vi "saveData.vi"(8 "error in (no error)":errorcluster, 11 "reference in":refnum<class "Devices Controller.lvclass">) -> (0 "error out":errorcluster, 3 "reference out":refnum<class "Devices Controller.lvclass">)   [LabVIEW 2016, in "Devices Controller.lvclass"]
uses:
  Devices Controller.lvclass
  APP/excelFile_class/fileType.ctl
  File Controller_llb/File Controller.lvclass
  APP/excelFile_class/excelFile.lvclass
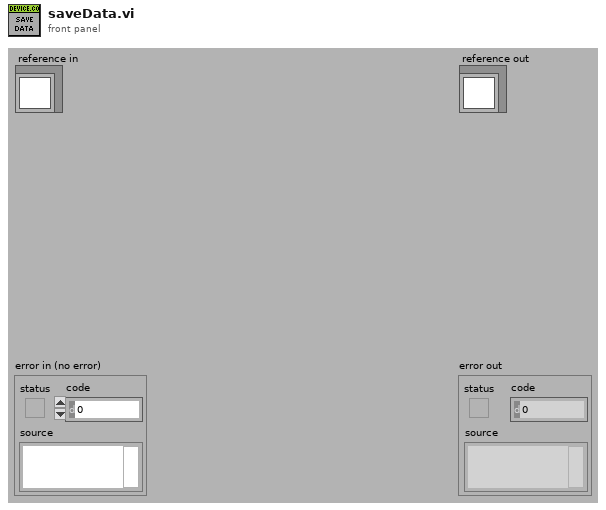
[diagram p1: front panel]
types:
  T1 = typedef "excelFile.lvclass/fileType.ctl" = enum16{"devices", "items", "partsTracking", "TSR"}
  T2 = typedef "Devices Controller.lvclass/ObjectAttributesRef.ctl" = refnum<data-value>
  T3 = typedef "Devices Controller.lvclass/ObjectAttributes.ctl" = cluster{"MyAttribute":dbl, "file_controller_ref":refnum<class "File Controller.lvclass">, "data":string[][][], "devices_refs":cluster{"k4b2_refs":refnum<class "k4b2.lvclass">[], "rmr_refs":refnum<class "rmr.lvclass">[], "bod_pod_refs":refnum<class "bodpod.lvclass">[], "cpet_refs":refnum<class "cpet.lvclass">[], "fitmate_refs":refnum<class "fitmate.lvclass">[], "pea_pod_refs":refnum<class "peapod.lvclass">[], "k5_refs":refnum<class "k5.lvclass">[], "bb-pft_refs":refnum<class "bb-pft.lvclass">[]}}
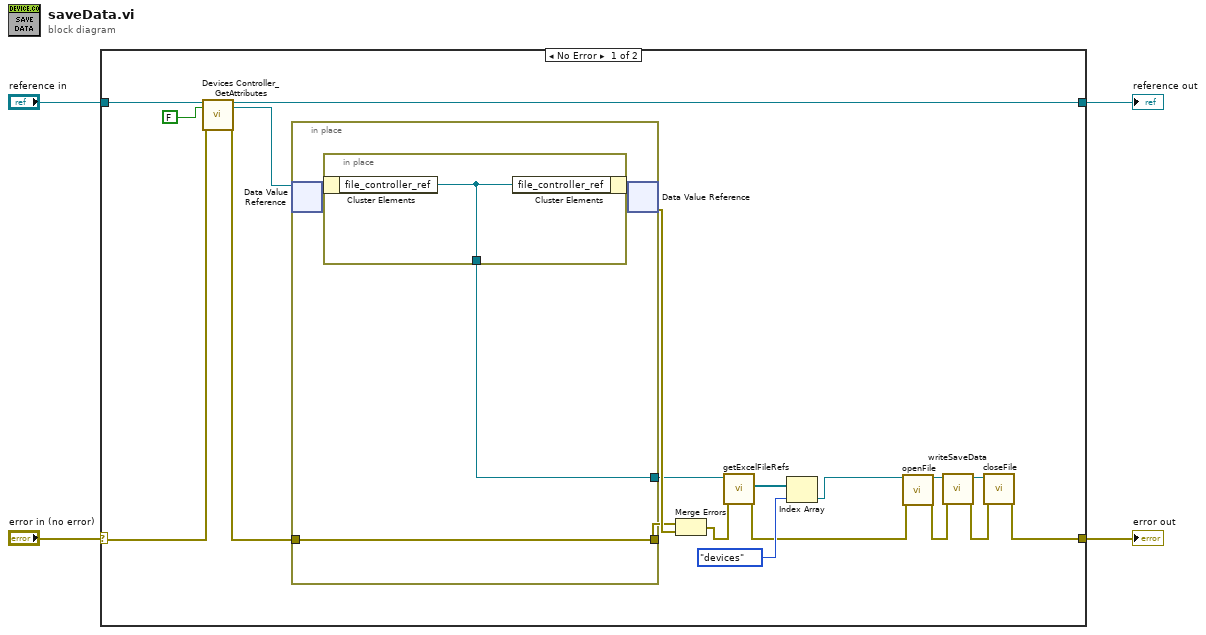
[diagram p0: block diagram]
diagram:
  n1 = case shown="No Error" "error in (no error)" {
    selector: "error in (no error)" -> [w19 w30]
    tunnel: [w11 w30] -> w3
    tunnel: [w17 w29] -> w1
    tunnel: "reference in" -> [w21 w29]
    frame No Error {
      n2 = call "Devices Controller_GetAttributes.vi"("reference in"=w21, "return data? (T)"=FALSE, "error in (no error)"=w19) -> ("reference out"=w17:refnum<class "Devices Controller.lvclass">, "attributes ref"=w16:T2, "error out"=w18:errorcluster)  [unwired: 13 in, 1 out]
      n3 = in-place {
        in-place-border: w18 -> [w25]
        in-place-border: [w25] -> w22
        in-place-border: [w24] -> w14
        n4 = in-place-dvr #1(w16) -> (w26:T3)  [unwired: 1 out]
        n5 = in-place {
          in-place-border: [w28] -> w24
          n6 = in-place-cluster #2(w26) -> ("file_controller_ref"=w28:refnum<class "File Controller.lvclass">)
          n7 = in-place-cluster #2("file_controller_ref"=w28) -> (w27:T3)
        }
        n8 = in-place-dvr #1(w27) -> (w23:errorcluster)  [unwired: 1 out]
      }
      n9 = Merge Errors(w22, w23) -> (w15:errorcluster)
      n10 = call "getExcelFileRefs.vi"("error in (no error)"=w15, "reference in"=w14) -> ("error out"=w6:errorcluster, "excelFile_refs"=w13:refnum<class "excelFile.lvclass">[])  [unwired: 7 in, 1 out]
      n11 = Index Array(array=w13, index=fileType."devices" ("fileType")) -> (element=w5:refnum<class "excelFile.lvclass">)
      n12 = call "openFile.vi"("reference in"=w5, "error in (no error)"=w6) -> ("reference out"=w8:refnum<class "excelFile.lvclass">, "error out"=w7:errorcluster)  [unwired: 16 in]
      n13 = call "writeSaveData.vi"("error in (no error)"=w7, "reference in"=w8) -> ("error out"=w9:errorcluster, "reference out"=w10:refnum<class "excelFile.lvclass">)  [unwired: 8 in]
      n14 = call "closeFile.vi"("error in (no error)"=w9, "reference in"=w10) -> ("error out"=w11:errorcluster)  [unwired: 8 in, 1 out]
    }
    frame Error {
    }
  }
  "error out" <- w3
  "reference out" <- w1
